vi "fileactionselector(SubVI).vi"(10 "Choose Update, Create, or Index File":string, 11 "String":string) -> (0 "error out":errorcluster, 3 "Byte Stream File out":refnum<file>)   [LabVIEW 2021]
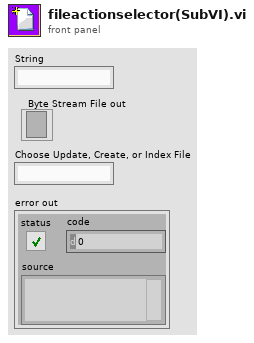
[diagram p1: front panel]
types:
  T1 = enum16{"open", "replace", "create", "open or create", "replace or create", "replace or create with confirmation"}
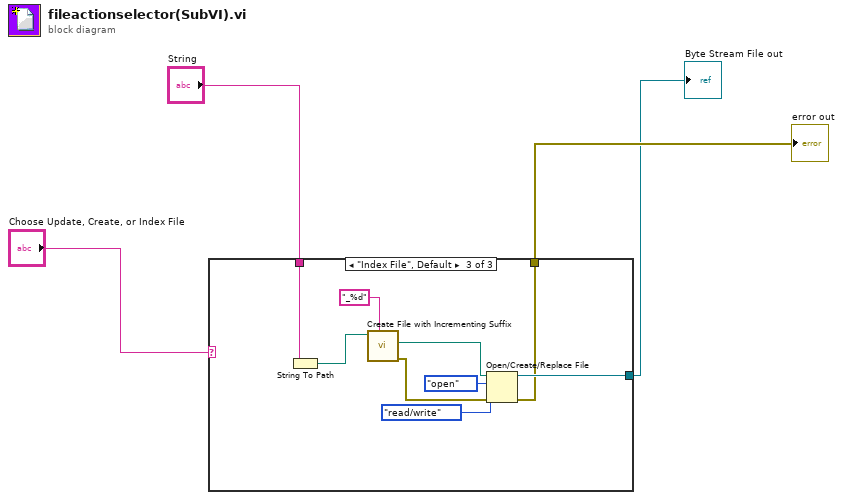
[diagram p0: block diagram]
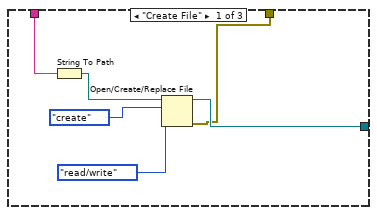
[diagram p2: hidden frame]
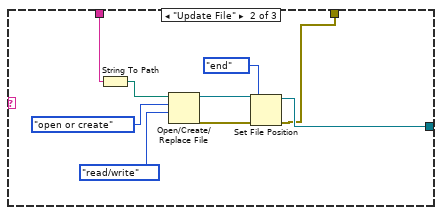
[diagram p3: hidden frame]
diagram:
  n1 = case shown="\"Index File\", Default" "Choose Update, Create, or Index File" {
    tunnel: [w10 w16 w24] -> w1
    tunnel: [w9 w14 w23] -> w2
    tunnel: "String" -> [w6 w19 w22]
    frame "Create File" {
      n2 = String To Path(string=w6) -> (path=w5:path)
      n3 = Open/Create/Replace File(file path (use dialog)=w5, operation (0:open)=T1."create", access (0:read/write)=enum16{"read/write", "read-only", "write-only"}."read/write") -> (refnum out=w10:refnum<file>, error out=w9:errorcluster)  [unwired: 3 in, 1 out]
    }
    frame "Update File" {
      n4 = String To Path(string=w19) -> (path=w18:path)
      n5 = Open/Create/Replace File(file path (use dialog)=w18, operation (0:open)=T1."open or create", access (0:read/write)=enum16{"read/write", "read-only", "write-only"}."read/write") -> (refnum out=w17:refnum<file>, error out=w13:errorcluster)  [unwired: 3 in, 1 out]
      n6 = Set File Position(refnum=w17, from (0:start)=enum16{"start", "end", "current"}."end", error in=w13) -> (refnum out=w16:refnum<file>, error out=w14:errorcluster)  [unwired: 1 in]
    }
    frame "Index File", Default {
      n7 = String To Path(string=w22) -> (path=w21:path)
      n8 = call <vilib>:"Create File with Incrementing Suffix.vi"("format string (\" (%d)\")"="_%d" ("format string (\" (%d)\")"), "file path"=w21) -> ("error out"=w20:errorcluster, "actual path"=w28:path)  [unwired: 7 in, 1 out]
      n9 = Open/Create/Replace File(file path (use dialog)=w28, error in=w20, operation (0:open)=T1."open", access (0:read/write)=enum16{"read/write", "read-only", "write-only"}."read/write") -> (refnum out=w24:refnum<file>, error out=w23:errorcluster)  [unwired: 2 in, 1 out]
    }
  }
  "error out" <- w2
  "Byte Stream File out" <- w1
